vi "INI_Driver.vi"(0 "Key":string, 1 "Config_File_Path":path, 2 "Section":string, 5 "Data_In":string, 11 "Error_Out":errorcluster, 13 "INI_Operation_Select":T1=enum."Write") -> (4 "Data_Out":string, 15 "Error_Out":errorcluster)   [LabVIEW 2021]
uses:
  <vilib>/Utility/config.llb/NI_LVConfig.lvlib
  <vilib>/Utility/config.llb/Read Key (String).vi
  <vilib>/Utility/config.llb/Write Key (String).vi
  Controls/INI_Operation_Select.ctl
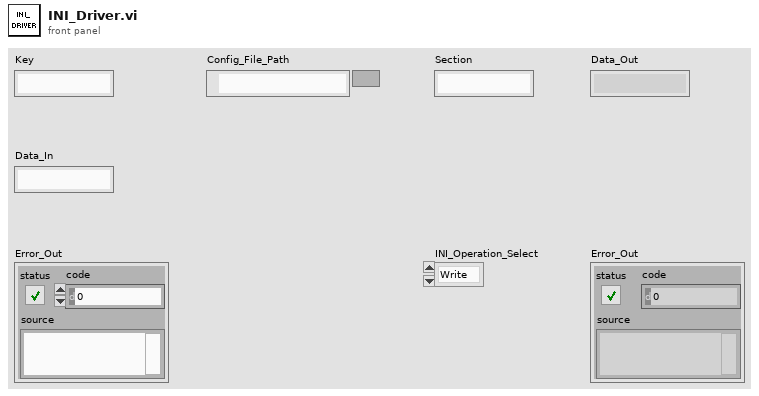
[diagram p1: front panel]
types:
  T1 = typedef "INI_Operation_Select.ctl" = enum16{"Initialize", "Read", "Write"}
  T2 = typedef "NI_LVConfig.lvlib/Config Data RefNum.ctl" = refnum<k1>
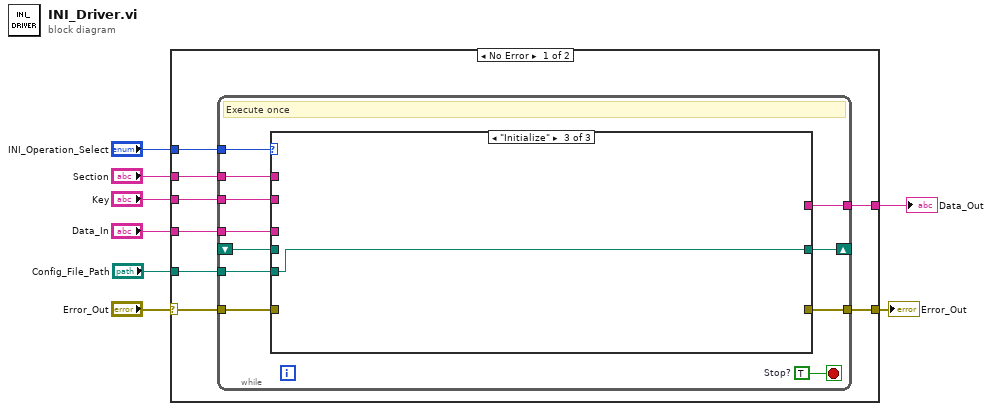
[diagram p0: block diagram]
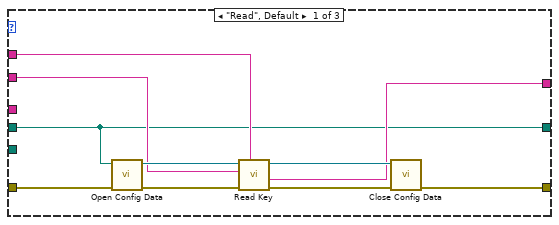
[diagram p2: hidden frame]
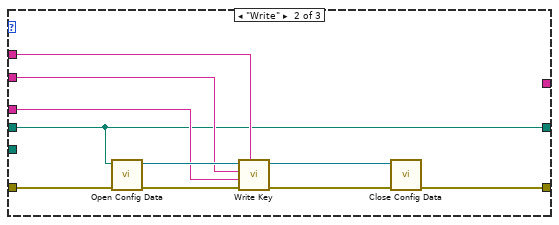
[diagram p3: hidden frame]
diagram:
  n1 = case shown="No Error" "Error_Out" {
    selector: "Error_Out" -> [w14 w49]
    tunnel: "INI_Operation_Select" -> [w16 _]
    tunnel: [w15 w49] -> w4
    tunnel: "Key" -> [w13 _]
    tunnel: "Section" -> [w12 _]
    tunnel: [w11 _] -> w3
    tunnel: "Data_In" -> [w10 _]
    tunnel: "Config_File_Path" -> [w9 _]
    frame No Error {
      n2 = while {
        tunnel: w16 -> [w27]
        tunnel: [w26] -> w15
        tunnel: w14 -> [w25]
        tunnel: w13 -> [w24]
        tunnel: w12 -> [w23]
        tunnel: [w21] -> w11
        tunnel: w10 -> [w20]
        shift-right: [w18] -> _
        shift-left: _ -> [w19]
        tunnel: w9 -> [w17]
        stop <- w22 stop-if-true
        w22 = TRUE  # Stop?
        # "Execute once"
        n3 = case shown="\"Initialize\"" w27 {
          tunnel: [w33 w43 _] -> w26
          tunnel: w25 -> [w37 w47 _]
          tunnel: w24 -> [w31 w41 _]
          tunnel: w23 -> [w30 w40 _]
          tunnel: [w29 _ _] -> w21
          tunnel: w20 -> [_ w39 _]
          tunnel: w19 -> [w28 w38 _]
          tunnel: [w28 w38 w48] -> w18
          tunnel: w17 -> [_ _ w48]
          frame "Read", Default {
            n4 = call <vilib>:"Open Config Data.vi"("error in (no error)"=w37, "configuration file path"=w28) -> ("error out"=w36:errorcluster, "refnum"=w35:T2)  [unwired: 7 in, 1 out]
            n5 = call-poly <vilib>:"Read Key.vi"("section"=w30, "error in (no error)"=w36, "key"=w31, "refnum"=w35) -> ("error out"=w34:errorcluster, "value"=w29:string, "refnum out"=w32:T2)  [unwired: 4 in, 1 out]
            n6 = call <vilib>:"Close Config Data.vi"("error in (no error)"=w34, "refnum"=w32) -> ("error out"=w33:errorcluster)  [unwired: 8 in, 1 out]
          }
          frame "Write" {
            n7 = call <vilib>:"Open Config Data.vi"("error in (no error)"=w47, "configuration file path"=w38) -> ("error out"=w46:errorcluster, "refnum"=w45:T2)  [unwired: 7 in, 1 out]
            n8 = call-poly <vilib>:"Write Key.vi"("section"=w40, "error in (no error)"=w46, "value"=w39, "key"=w41, "refnum"=w45) -> ("error out"=w44:errorcluster, "refnum out"=w42:T2)  [unwired: 4 in, 1 out]
            n9 = call <vilib>:"Close Config Data.vi"("error in (no error)"=w44, "refnum"=w42) -> ("error out"=w43:errorcluster)  [unwired: 8 in, 1 out]
          }
          frame "Initialize" {
          }
        }
      }
    }
    frame Error {
    }
  }
  "Error_Out" <- w4
  "Data_Out" <- w3
